vi "Delete All Springboards.vi"   [LabVIEW 2016]
panel:
  # "Removing All Springboards..."
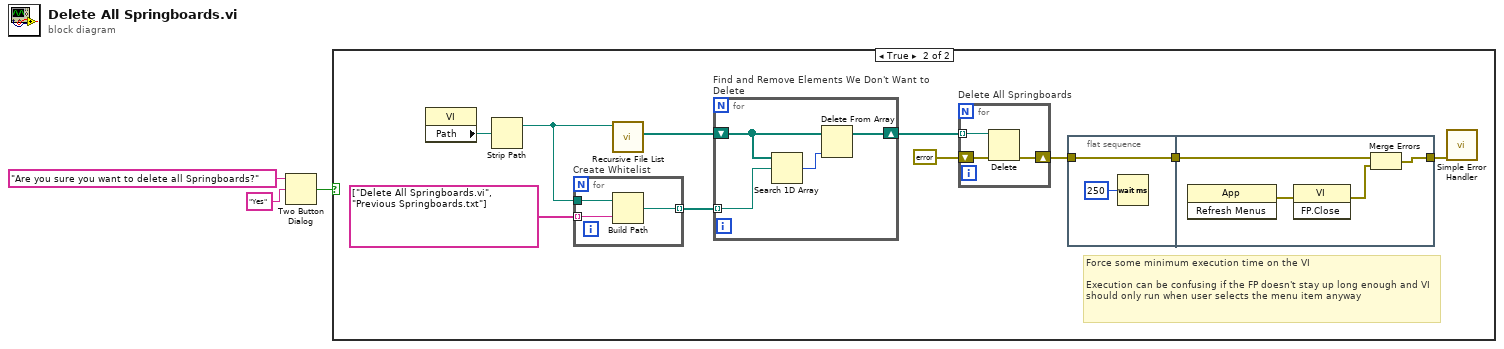
[diagram p0: block diagram]
diagram:
  n1 = Two Button Dialog(message="Are you sure you want to delete all Springboards?", 2:"Yes" ("T button name (\"OK\")")) -> (T button?=w3:bool)  [unwired: 1 in]
  n2 = case shown="True" w3 {
    frame False {
    }
    frame True {
      # "Force some minimum execution time on the VI\n\nExecution can be confusing if the FP doesn't stay up long enough and VI should only run when user selects the menu item anyway"
      n3 = property class="VI"() -> ("Path"=w12:path)  [unwired: 2 in, 2 out]
      n4 = Strip Path(path=w12) -> (stripped path=w6:path)  [unwired: 1 out]
      n5 = for "Create Whitelist" {
        tunnel: w6 -> [w16]
        tunnel: [w15] -> w5 mode=indexing
        tunnel: string[] ["Delete All Springboards.vi", "Previous Springboards.txt"] -> [w14] mode=indexing
        n6 = Build Path(base path=w16, name or relative path=w14) -> (appended path=w15:path)
      }
      n7 = call <vilib>:"Recursive File List.vi"("Folder Path"=w6) -> ("All Files in Dir"=w11:path[])  [unwired: 6 in, 4 out]
      n8 = for "Find and Remove Elements We Don't Want to Delete" {
        tunnel: w5 -> [w29] mode=indexing
        shift-right: [w27] -> w10
        shift-left: w11 -> [w28]
        n9 = Search 1D Array(1D array=w28, element=w29) -> (index of element=w26:i32)  [unwired: 1 in]
        n10 = Delete From Array(array=w28, index=w26) -> (array with subset deleted=w27:path[])  [unwired: 1 in, 1 out]
      }
      n11 = for "Delete All Springboards" {
        tunnel: w10 -> [w25] mode=indexing
        shift-right: [w24] -> w8
        shift-left: errorcluster {"status"=FALSE, "code"=0, "source"=""} ("error out") -> [w23]
        n12 = Delete(path (use dialog)=w25, error in=w23) -> (error out=w24:errorcluster)  [unwired: 3 in, 2 out]
      }
      n13 = flat-sequence {
        tunnel: w8 -> [w18]
        tunnel: [w18] -> w13
        tunnel: [w20] -> w7
        tunnel: w13 -> [w22]
        frame #0 {
          n14 = Wait (ms)(milliseconds to wait=u32 250) -> ()  [unwired: 1 out]
        }
        frame #1 {
          n15 = invoke class="App" method="Refresh Menus"() -> (error out=w21:errorcluster)  [unwired: 3 in, 2 out]
          n16 = invoke class="VI" method="FP.Close"(error in=w21) -> (error out=w19:errorcluster)  [unwired: 2 in, 2 out]
          n17 = Merge Errors(w22, w19) -> (w20:errorcluster)
        }
      }
      n18 = call <vilib>:"Simple Error Handler.vi"("error in (no error)"=w7) -> ()  [unwired: 4 in, 5 out]
    }
  }
